vi "Tester.vi"() -> ()   [LabVIEW 2013]
uses:
  Spark API.lvlib
panel:
  out "Function Response 2":T1
  in  "Code":string
  out "Function Response":T1
  out "Variable Response":string
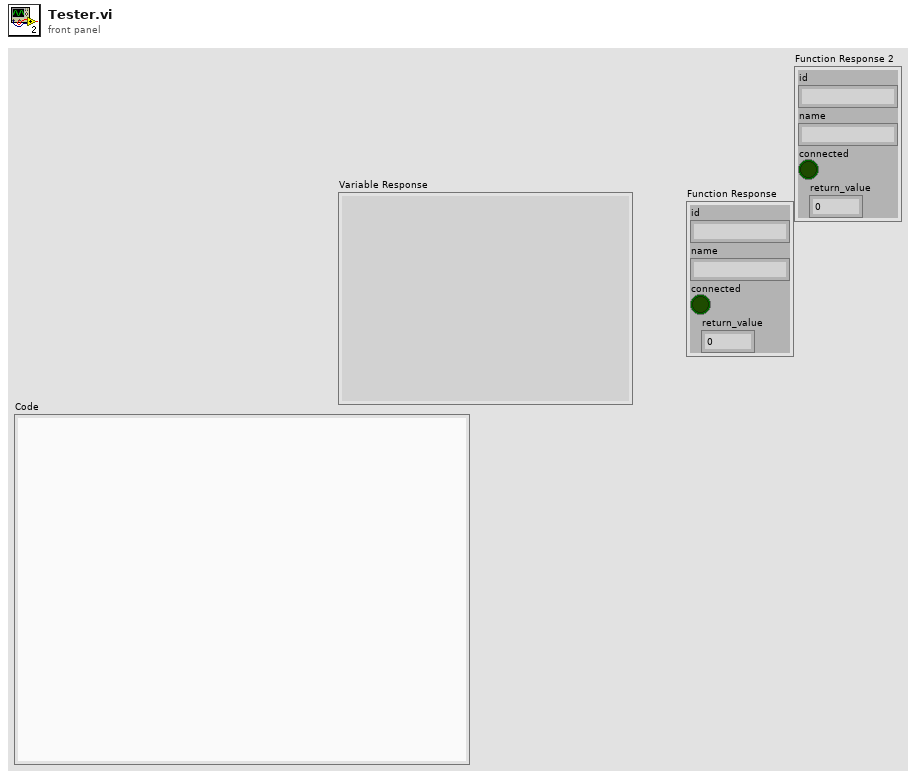
[diagram p1: front panel]
types:
  T1 = cluster{"id":string, "name":string, "connected":bool, "return_value":dbl}
  T2 = typedef "Spark API.lvlib/Spark Reference.ctl" = cluster{"client handle out":T3, "Access Token":string, "Device ID":string, "Device Query JSON":T4}
  T3 = typedef "LabVIEWHTTPClient.lvlib/ClientHandle.ctl" = refnum<k1>
  T4 = typedef "Spark API.lvlib/Device Query JSON.ctl" = cluster{"id":string, "name":string, "variables":string[], "functions":string[]}
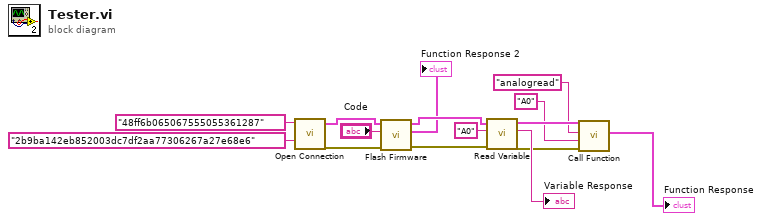
[diagram p0: block diagram]
diagram:
  n1 = call "Open Connection.vi"("Access Token"="2b9ba142eb852003dc7df2aa77306267a27e68e6", "Device ID"="48ff6b065067555055361287") -> ("error out"=w4:errorcluster, "Spark Reference"=w5:T2)  [unwired: 8 in]
  n2 = call "Flash Firmware.vi"("error in"=w4, "Code"="Code", "Spark Reference In"=w5) -> ("error out"=w2:errorcluster, "Function Response"=→"Function Response 2":T1, "Spark Reference Out"=w3:T2)  [unwired: 6 in]
  n3 = call "Read Variable.vi"("error in"=w2, "Variable Name"="A0", "Spark Reference In"=w3) -> ("error out"=w10:errorcluster, "Variable Response"=→"Variable Response":string, "Spark Reference Out"=w11:T2)  [unwired: 6 in]
  n4 = call "Call Function.vi"("error in"=w10, "Arguments"="A0", "Function Name"="analogread", "Spark Reference In"=w11) -> ("Function Response"=→"Function Response":T1)  [unwired: 5 in, 2 out]
